vi "qTAD.vi"(0 "System no.":i32=1 min=1 max=4 step=1, 2 "Sensor to query":string[](array[string]), 3 "All sensors?":bool, 4 "Sensor identifier?":bool=TRUE, 5 "error in":errorcluster) -> (14 "AD value":dbl[](array[numeric]) format="%.6f", 15 "Sensors to query out":string[](array[string]), 19 "error out":errorcluster)   [LabVIEW 2026]
doc: "Returns AD value for the specified sensor number.\n\nC-413 : If All sensors? = TRUE, then Sensor identifier? must be FALSE. Sensors to query comprises all ADC channels of the device: can be a \"genuine\" sensor (sensor integrated in the mechanics) or a \"general purpose\" analog input.\n\nE-517, E-518: If All sensors? = TRUE, then Sensor identifier? must be FALSE. The input signal channels to be queried with TAD? are the sensor channels of the piezo control electronics, IDs = 1 to 3 (actually available IDs depend on the response to TSC?).\n\nE-709: If All sensors? = TRUE, then Sensor identifier? must be FALSE. Sensors to query comprises all ADC channels of the device: can be the \"genuine\" sensor (sensor integrated in the mechanics, identifier = 1) and the \"general purpose\" analog input (identifier = 2).\n\nE-710: If All sensors? = TRUE, then Sensor identifier? must be TRUE. Command is available for 4-channel controller only and in command level 1 only (see CCL.vi and CCL?.vi)\n\nE-712: If All sensors? = TRUE, then Sensor identifier? must be FALSE. Sensors to query comprises all ADC channels of the device: can be a \"genuine\" sensor (sensor integrated in the mechanics) or a \"general purpose\" analog input.\n\nE-725, E-727: If All sensors? = TRUE, then Sensor identifier? must be FALSE. Sensors to query comprises all ADC channels of the device: can be a \"genuine\" sensor (sensor integrated in the mechanics) or a \"general purpose\" analog input.\n\nE-753: If All sensors? = TRUE, then Sensor identifier? must be FALSE. Sensors to query comprises all ADC channels of the device: can be the \"genuine\" sensor (capacitive sensor integrated in the mechanics, identifier = 1) and the \"general purpose\" analog input (identifier = 2).\n\nE-754: If All sensors? = TRUE, then Sensor identifier? must be FALSE. Sensors to query comprises all ADC channels of the device: can be the \"genuine\" sensor (capacitive sensor integrated in the mechanics, identifier = 1, or incremental sensor, identifier = 3) and the \"general purpose\" analog input (identifier = 2).\n\nE-755: If All sensors? = TRUE, then Sensor identifier? must be FALSE. Command not available for E-755.101.\n\nE-761: Sensors to query can be 1 to 3. If All sensors? = TRUE, then Sensor identifier? can be FALSE.\n\nE-870: Sensors to query comprises all ADC channels of the device: can be the analog command input (identifier = 1) or other internal on board sources for diagnosis information (identifier = 2…5).\n\nC-887, F-206, M-8X0: If All sensors? = TRUE, then Sensor identifier? must be FALSE. Only for GCS syntax version = GCS 2.0 or higher (check with CSV?.vi. If CSV?.vi is not supported, syntax version is GCS 1.0)."
panel:
  # "Returns AD value for the specified sensor number."
  # "If all sensors: use"
  # "Query"
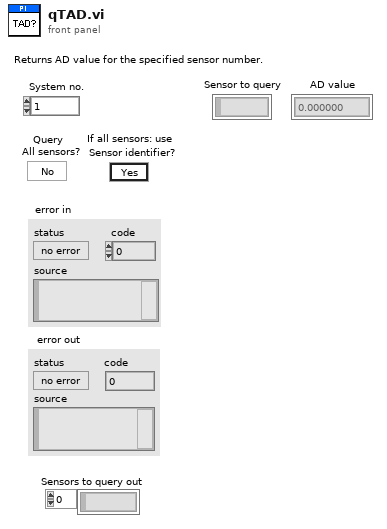
[diagram p1: front panel]
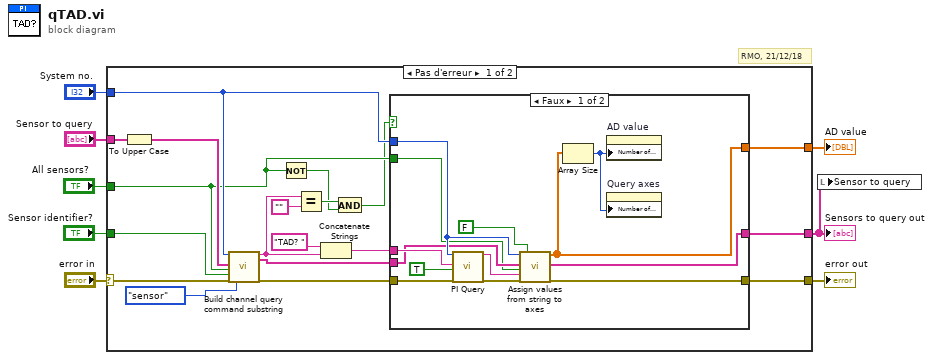
[diagram p0: block diagram]
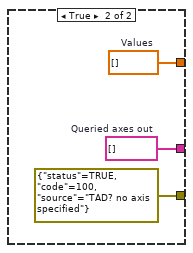
[diagram p2: hidden frame]
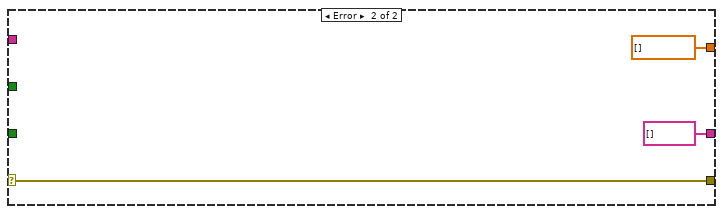
[diagram p3: hidden frame]
diagram:
  # "RMO, 21/12/18"
  n1 = case shown="Pas d'erreur" "error in" {
    selector: "error in" -> [w11 w44]
    tunnel: [w14 dbl[] [] ("Values")] -> w8
    tunnel: "Sensor to query" -> [w25 _]
    tunnel: [w10 w44] -> w6
    tunnel: "Sensor identifier?" -> [w16 _]
    tunnel: "System no." -> [w20 _]
    tunnel: "All sensors?" -> [w12 _]
    tunnel: [w13 string[] [] ("Queried axes out")] -> w2
    frame No Error {
      n2 = To Upper Case(1:w25) -> (0:w17:string[])
      n3 = call "Build channel query command substring.vi"("System no."=w20, "Channels to query in"=w17, "Query\nAll channels?"=w12, "For all channels: use\nChannel identifier?"=w16, "error in"=w11, "Channel type"=enum16{"piezo", "sensor"}."sensor") -> ("Command substring"=w19:string, "Channels to query out"=w15:string[], "error out"=w18:errorcluster)  [unwired: 1 in, 10 out]
      n4 = Not(x=w12) -> (.not. x?=w22:bool)
      n5 = Equal?(x=w19, y="" ("x")) -> (x = y?=w23:bool)
      n6 = Concatenate Strings("TAD? ", w19) -> (w26:string)
      n7 = And(x=w23, y=w22) -> (x .and. y?=w9:bool)
      n8 = case shown="Faux" w9 {
        tunnel: w26 -> [w39 _]
        tunnel: w20 -> [w38 _]
        tunnel: w18 -> [w37 _]
        tunnel: w15 -> [w36 _]
        tunnel: [w35 w43] -> w14
        tunnel: [w33 w42] -> w13
        tunnel: w12 -> [w32 _]
        tunnel: [w30 errorcluster {"status"=TRUE, "code"=100, "source"="TAD? no axis specified"} ("error out")] -> w10
        frame False {
          n9 = call "PI Query.vi"("System no."=w38, "String to send"=w39, "Attach termination char.?"=TRUE ("Attach Linefeed?"), "error in"=w37) -> ("String read"=w28:string, "error out"=w29:errorcluster)  [unwired: 3 in, 11 out]
          n10 = call "Assign values from string to axes.vi"("System no."=w38, "Queried axes"=w36, "All axes queried?"=w32, "Input String"=w28, "error in"=w29, "Axes related?"=FALSE) -> ("Values"=w35:dbl[], "Queried axes out"=w33:string[], "error out"=w30:errorcluster)  [unwired: 3 in, 8 out]
          n11 = Array Size(array=w35) -> (size(s)=w34:i32)
          n12 = property on="AD value" class="Tabl (strict)"("Number of Rows"=w34) -> ()  [unwired: 2 in, 2 out]
          n13 = property on="Query axes" class="Tabl (strict)"("Number of Rows"=w34) -> ()  [unwired: 2 in, 2 out]
        }
        frame True {
          w42 = string[] []  # Queried axes out
          w43 = dbl[] []  # Values
        }
      }
    }
    frame Error {
    }
  }
  "error out" <- w6
  "AD value" <- w8
  "Sensors to query out" <- w2
  n14 = local write "Sensor to query"(w2) -> ()
